vi "GetDO.vi"(9 "select":u8, 10 "sn":string) -> (2 "output frame":string)   [LabVIEW 2012]
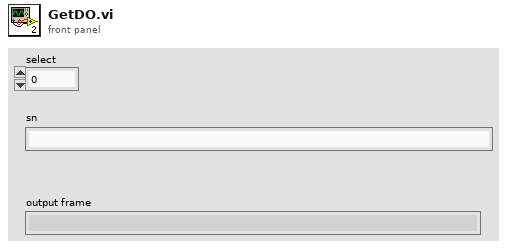
[diagram p1: front panel]
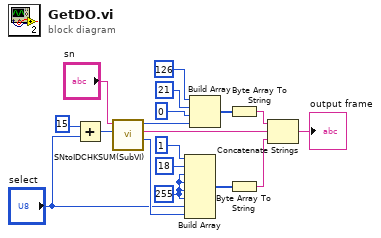
[diagram p0: block diagram]
diagram:
  w18 = u8 255
  n1 = Add(x=u8 15, y="select") -> (x+y=w3:u8)
  n2 = call "SNtoIDCHKSUM(SubVI).vi"("fix cheksum"=w3, "input sn"="sn") -> ("output check sum"=w2:u8, "output sn"=w14:string, "output id"=w7:u8)  [unwired: 7 in]
  n3 = Build Array(u8 1, u8 18, w18, w18, w18, w18, "select", w2) -> (w11:u8[])
  n4 = Build Array(u8 126, u8 21, u8 0, w7) -> (w12:u8[])
  n5 = Byte Array To String(unsigned byte array=w12) -> (string=w13:string)
  n6 = Byte Array To String(unsigned byte array=w11) -> (string=w15:string)
  n7 = Concatenate Strings(w13, w14, w15) -> (→"output frame":string)
